vi "Relay Set (Tank Fill).vi"(8 "error in (no error)":errorcluster, 10 "RelayValue":enum16{"Off", "On"}(ring), 11 "RelayDevRef":cluster{string, i32}) -> (0 "error out":errorcluster, 3 "RelayDevRef":cluster{string, i32})   [LabVIEW 2013]
uses:
  Tank Fill Global.vi
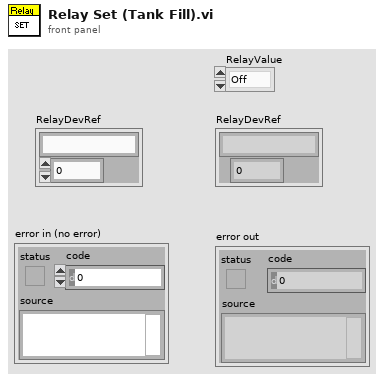
[diagram p1: front panel]
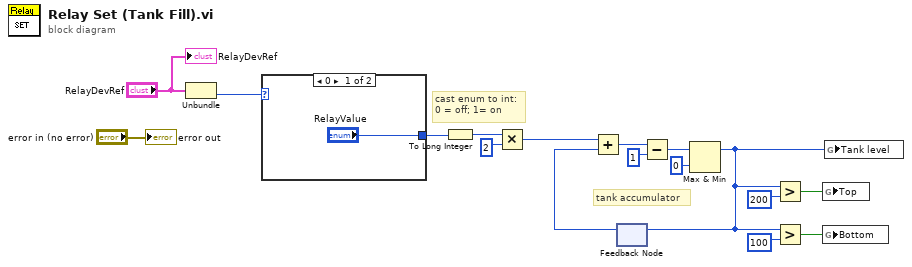
[diagram p0: block diagram]
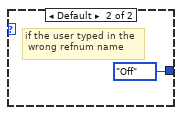
[diagram p2: hidden frame]
diagram:
  # "cast enum to int:\n0 = off; 1= on"
  # "tank accumulator"
  n1 = Unbundle("RelayDevRef") -> (w15:i32)  [unwired: 1 out]
  n2 = case shown="0" w15 {
    tunnel: ["RelayValue" enum16{"Off", "On"}."Off" ("RelayValue")] -> w14
    frame 0 {
    }
    frame Default {
      # "if the user typed in the\n wrong refnum name"
    }
  }
  n3 = To Long Integer(number=w14) -> (32bit integer=w13:i32)
  n4 = Multiply(x=w13, y=2) -> (x*y=w11:i32)
  n5 = feedback #1() -> (w10:i32)  [unwired: 1 in]
  n6 = Add(x=w11, y=w10) -> (x+y=w5:i32)
  n7 = Subtract(x=w5, y=1) -> (x-y=w3:i32)
  n8 = Max & Min(x=w3, y=0) -> (max(x,y)=w2:i32)  [unwired: 1 out]
  n9 = feedback-in #1(w2) -> ()
  n10 = Greater?(x=w2, y=200) -> (0:w7:bool)
  n11 = Greater?(x=w2, y=100) -> (0:w6:bool)
  n12 = global write "Tank Fill Global.vi" "Top"(w7) -> ()
  n13 = global write "Tank Fill Global.vi" "Bottom"(w6) -> ()
  n14 = global write "Tank Fill Global.vi" "Tank level"(w2) -> ()
  "error out" <- "error in (no error)"
  "RelayDevRef" <- "RelayDevRef"
